vi "DB5000.X写 -AllRest.vi"(0 "引用":refnum<k24>, 5 "semaphore":T1 caption="信号量", 7 "地址名称":string(combo)="字符识别启动信号-读", 11 "error in (no error)":errorcluster caption="错误输入（无错误）") -> (4 "引用输出":refnum<k24>, 15 "error out":errorcluster caption="错误输出")   [LabVIEW 2017]
panel:
  # "字符识别启动信号-读                 DB5000,X00\n电脑1扫码枪触发-读                  DB5000,X100\n电脑1CCD读取字符触发-读         DB5000.101\n电脑1表面检测触发-读               DB5000.102\n电脑1穿管检测触发-读               DB5000.103\n区间位置1-读       DB5000.104\n区间位置2-读       DB5000.105\n区间位置3-读       DB5000.106\n区间位置4-读       DB5000.107\n区间位置5-读       DB5000.108\n区间位置6-读       DB5000.109\n区间位置7-读       DB5000.110\n区间位置8-读       DB5000.111\n区间位置9-读       DB5000.112\n区间位置10-读     DB5000.113\n区间位置11-读      DB5000.114\n区间位置12-读      DB5000.115\n区间位置13-读      DB5000.116\n区间位置14-读      DB5000.117\n区间位置15-读      DB5000.118\n区间位置16-读      DB5000.119\n区间位置17-读      DB5000.120\n区间位置18-读      DB5000.121\n区间位置19-读      DB5000.122\n夹爪1状态-读        DB5000.123\n夹爪2状态-读        DB5000.124\n夹爪3状态-读        DB5000.125\n夹爪4状态-读        DB5000.126\n夹爪5状态-读        DB5000.127\n夹爪6状态-读        DB5000.128\n夹爪7状态-读        DB5000.129\n夹爪8状态-读        DB5000.130\n夹爪9状态-读        DB5000.131\n夹爪10状态-读      DB5000.132\n电脑1产品前后位置切换触发-读       DB5000.133\n电脑1压力获取触发-读                    DB5000.134\nPC1 ready-写                       DB5000.200\n混料-写                               DB5000.201\n字符1检测pass-写                DB5000.202\n字符1检测fail-写                  DB5000.203\n表面检测pass-写                 DB5000.204\n表面检测fail-写                    DB5000.205\n穿管检测pass-写                 DB5000.206\n穿管检测fail-写                    DB5000.207\n扫码枪pass-写                     DB5000.208\n扫码枪fail-写                       DB5000.209\n产品尺寸A-写                      DB5000.210\n产品尺寸B-写                       DB5000.211\n数据传递信号-读                  DB5000.212\n表面检测完成信号-读             DB5000.213\n穿管NG停止信号-写              DB5000.214\n电脑1返工信号-写                 DB5000.215\nPLC初始化信号-读                DB5000.216\n产品尺寸C-写                       DB5000.217\n表面检测错位气缸-读             DB5000.218   \n电脑1衬丝检测触发-读           DB5000.219\n衬丝能检测pass-写               DB5000.220\n衬丝能检测fail-写                  DB5000.221\n长衬丝-写                            DB5000.222\n短衬丝-写                            DB5000.223\n细料-写                              DB5000.225\n粗料-写                              DB5000.226\n一致性检测触发-读               DB5000.227"
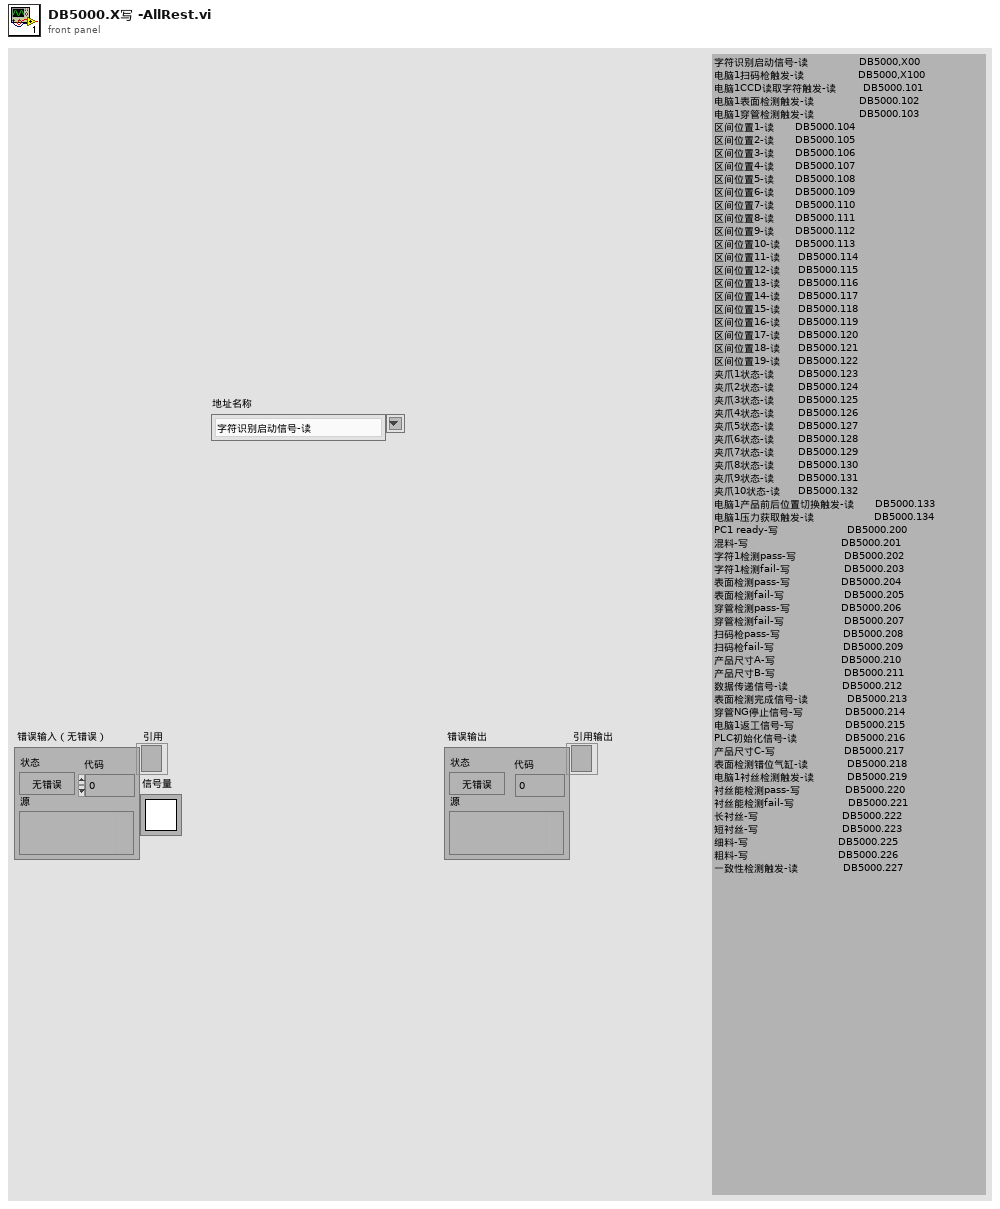
[diagram p1: front panel]
types:
  T1 = typedef "Semaphore RefNum" = refnum<k1>
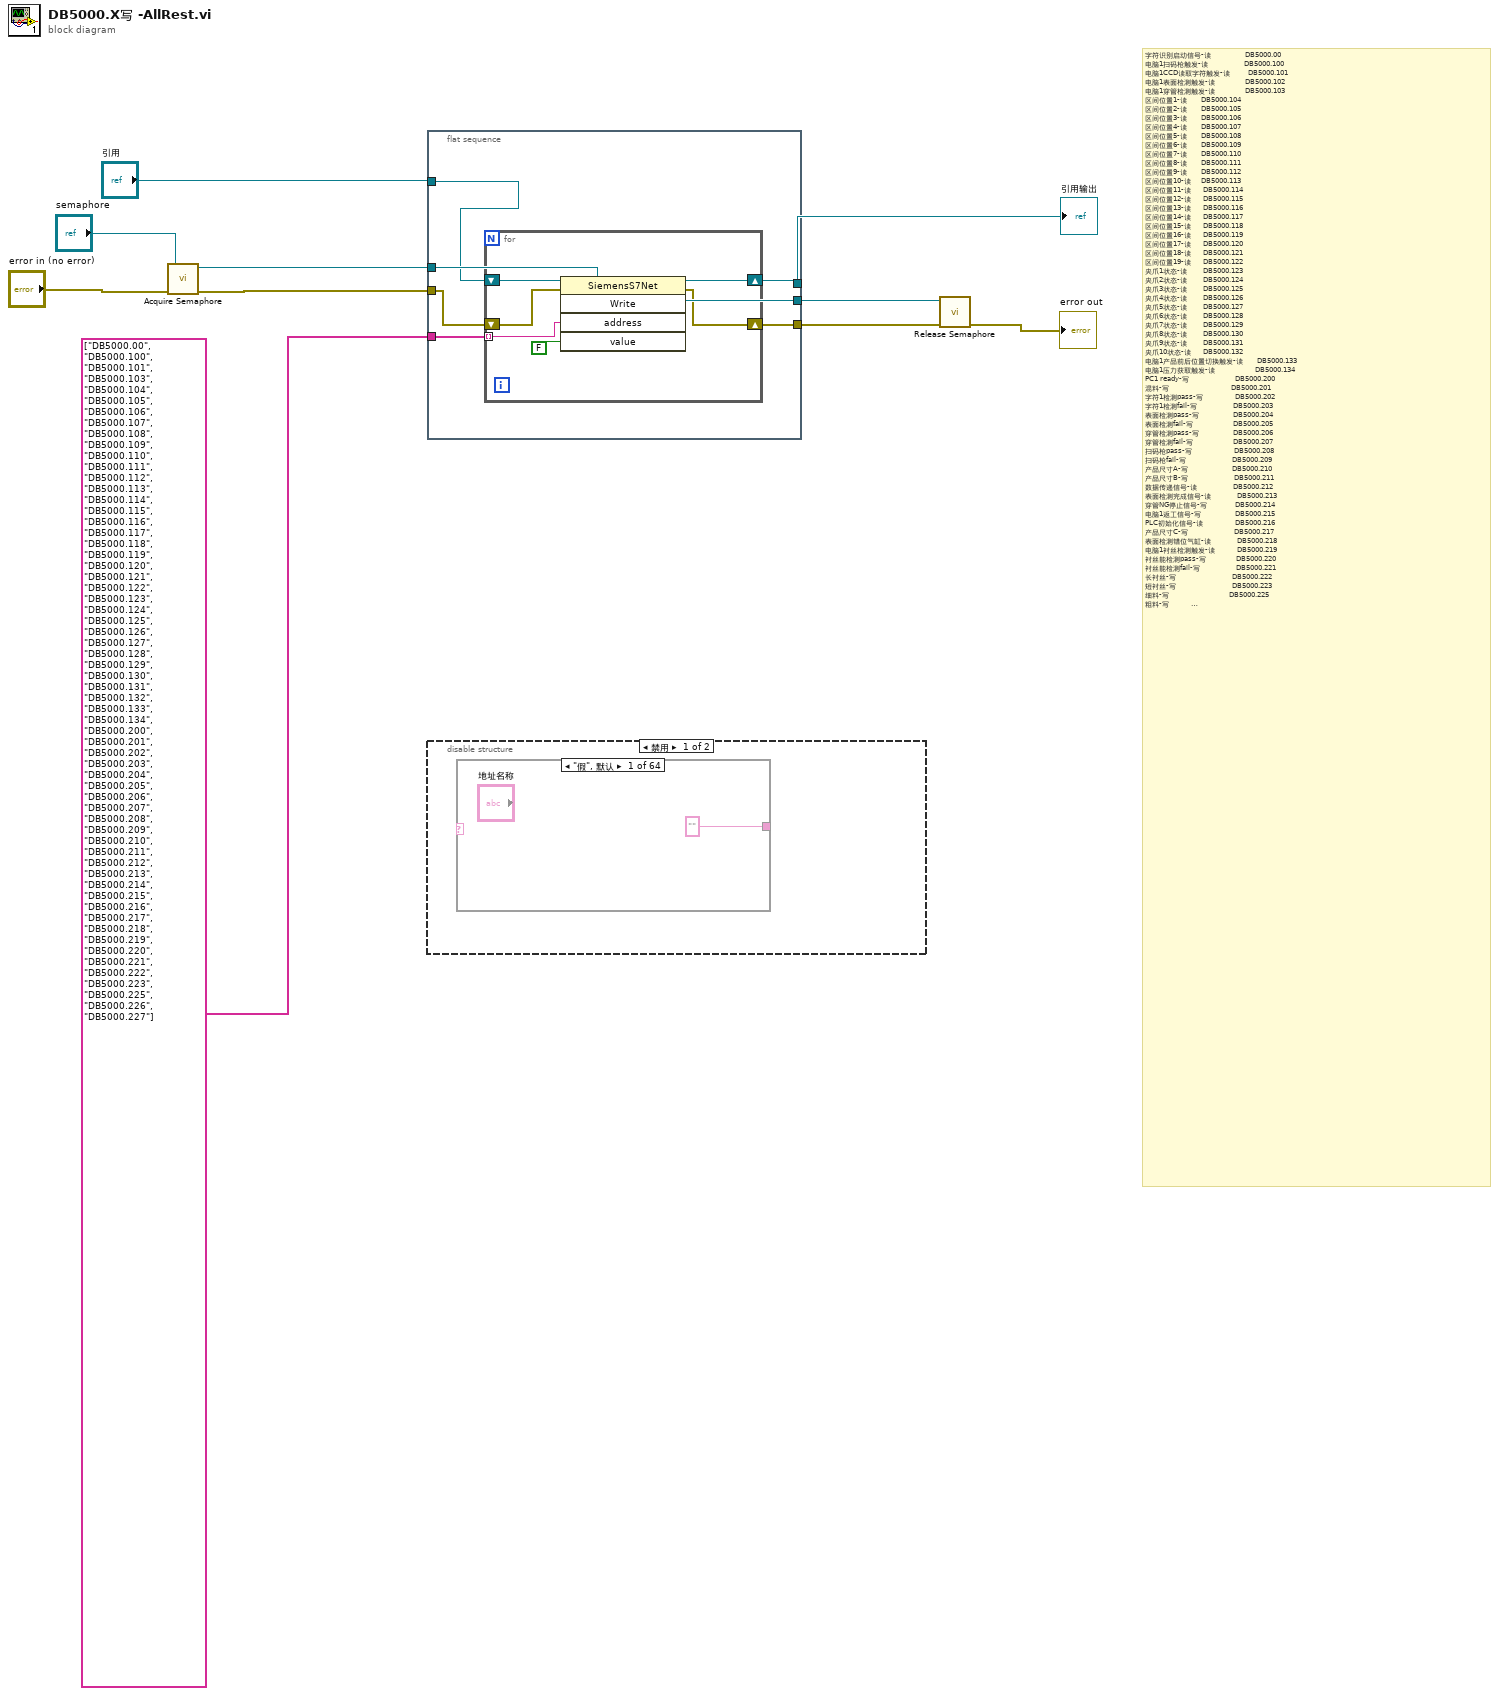
[diagram p0: block diagram]
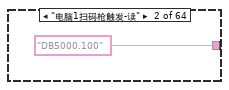
[diagram p2: hidden frame]
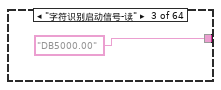
[diagram p3: hidden frame]
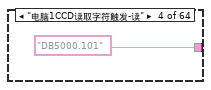
[diagram p4: hidden frame]
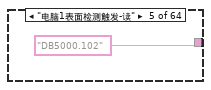
[diagram p5: hidden frame]
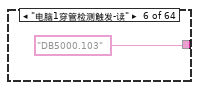
[diagram p6: hidden frame]
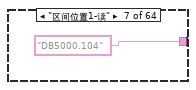
[diagram p7: hidden frame]
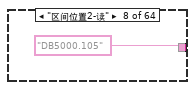
[diagram p8: hidden frame]
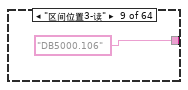
[diagram p9: hidden frame]
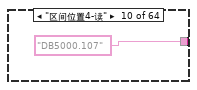
[diagram p10: hidden frame]
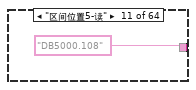
[diagram p11: hidden frame]
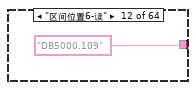
[diagram p12: hidden frame]
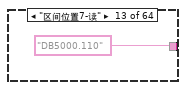
[diagram p13: hidden frame]
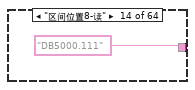
[diagram p14: hidden frame]
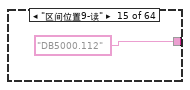
[diagram p15: hidden frame]
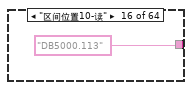
[diagram p16: hidden frame]
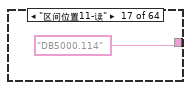
[diagram p17: hidden frame]
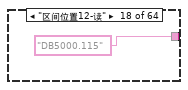
[diagram p18: hidden frame]
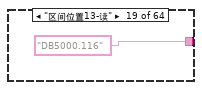
[diagram p19: hidden frame]
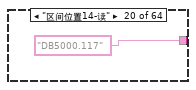
[diagram p20: hidden frame]
diagram:
  # "字符识别启动信号-读                 DB5000.00\n电脑1扫码枪触发-读                  DB5000.100\n电脑1CCD读取字符触发-读         DB5000.101\n电脑1表面检测触发-读               DB5000.102\n电脑1穿管检测触发-读               DB5000.103\n区间位置1-读       DB5000.104\n区间位置2-读       DB5000.105\n区间位置3-读       DB5000.106\n区间位置4-读       DB5000.107\n区间位置5-读       DB5000.108\n区间位置6-读       DB5000.109\n区间位置7-读       DB5000.110\n区间位置8-读       DB5000.111\n区间位置9-读       DB5000.112\n区间位置10-读     DB5000.113\n区间位置11-读      DB5000.114\n区间位置12-读      DB5000.115\n区间位置13-读      DB5000.116\n区间位置14-读      DB5000.117\n区间位置15-读      DB5000.118\n区间位置16-读      DB5000.119\n区间位置17-读      DB5000.120\n区间位置18-读      DB5000.121\n区间位置19-读      DB5000.122\n夹爪1状态-读        DB5000.123\n夹爪2状态-读        DB5000.124\n夹爪3状态-读        DB5000.125\n夹爪4状态-读        DB5000.126\n夹爪5状态-读        DB5000.127\n夹爪6状态-读        DB5000.128\n夹爪7状态-读        DB5000.129\n夹爪8状态-读        DB5000.130\n夹爪9状态-读        DB5000.131\n夹爪10状态-读      DB5000.132\n电脑1产品前后位置切换触发-读       DB5000.133\n电脑1压力获取触发-读                    DB5000.134\nPC1 ready-写                       DB5000.200\n混料-写                               DB5000.201\n字符1检测pass-写                DB5000.202\n字符1检测fail-写                  DB5000.203\n表面检测pass-写                 DB5000.204\n表面检测fail-写                    DB5000.205\n穿管检测pass-写                 DB5000.206\n穿管检测fail-写                    DB5000.207\n扫码枪pass-写                     DB5000.208\n扫码枪fail-写                       DB5000.209\n产品尺寸A-写                      DB5000.210\n产品尺寸B-写                       DB5000.211\n数据传递信号-读                  DB5000.212\n表面检测完成信号-读             DB5000.213\n穿管NG停止信号-写              DB5000.214\n电脑1返工信号-写                 DB5000.215\nPLC初始化信号-读                DB5000.216\n产品尺寸C-写                       DB5000.217\n表面检测错位气缸-读             DB5000.218   \n电脑1衬丝检测触发-读           DB5000.219\n衬丝能检测pass-写               DB5000.220\n衬丝能检测fail-写                  DB5000.221\n长衬丝-写                            DB5000.222\n短衬丝-写                            DB5000.223\n细料-写                              DB5000.225\n粗料-写                              DB5000.226\n一致性检测触发-读               DB5000.227"
  n1 = call <vilib>:"Acquire Semaphore.vi"("error in (no error)"="error in (no error)", "semaphore"="semaphore") -> ("error out"=w9:errorcluster, "semaphore out"=w7:T1)  [unwired: 3 in, 1 out]
  n2 = flat-sequence {
    tunnel: [w16] -> w10
    tunnel: w9 -> [w15]
    tunnel: [w14] -> w8
    tunnel: w7 -> [w14]
    tunnel: "引用" -> [w13]
    tunnel: [w12] -> w2
    tunnel: string[] ["DB5000.00", "DB5000.100", "DB5000.101", "DB5000.103", "DB5000.104", "DB5000.105", "DB5000.106", "DB5000.107", "DB5000.108", "DB5000.109", "DB5000.110", "DB5000.111", "DB5000.112", "DB5000.113", "DB5000.114", "DB5000.115", "DB5000.116", "DB5000.117", "DB5000.118", "DB5000.119", "DB5000.120", "DB5000.121", "DB5000.122", "DB5000.123", "DB5000.124", "DB5000.125", "DB5000.126", "DB5000.127", "DB5000.128", "DB5000.129", "DB5000.130", "DB5000.131", "DB5000.132", "DB5000.133", "DB5000.134", "DB5000.200", "DB5000.201", "DB5000.202", "DB5000.203", "DB5000.204", "DB5000.205", "DB5000.206", "DB5000.207", "DB5000.208", "DB5000.209", "DB5000.210", "DB5000.211", "DB5000.212", "DB5000.213", "DB5000.214", "DB5000.215", "DB5000.216", "DB5000.217", "DB5000.218", "DB5000.219", "DB5000.220", "DB5000.221", "DB5000.222", "DB5000.223", "DB5000.225", "DB5000.226", "DB5000.227"] -> [w11]
    frame #0 {
      n3 = for {
        shift-right: [w22] -> w16
        shift-left: w15 -> [w21]
        shift-right: [w19] -> w12
        shift-left: w13 -> [w20]
        tunnel: w11 -> [w17] mode=indexing
        n4 = invoke class="SiemensS7Net" method="Write"(reference=w20, error in=w21, "address"=w17, "value"=FALSE) -> (reference out=w19:refnum<k24>, error out=w22:errorcluster)  [unwired: 1 in, 3 out]
      }
    }
  }
  n5 = disable-structure shown="禁用" {
    frame Disabled {
      n6 = case shown="\"假\", 默认" {
        selector: _ -> [_ _ _ _ _ _ _ _ _ _ _ _ _ _ _ _ _ _ _ _ _ _ _ _ _ _ _ _ _ _ _ _ _ _ _ _ _ _ _ _ _ _ _ _ _ _ _ _ _ _ _ _ _ _ _ _ _ _ _ _ _ _ _ _]
        tunnel: ["" ("组合框") "DB5000.100" ("组合框") "DB5000.00" ("组合框") "DB5000.101" ("组合框") "DB5000.102" ("组合框") "DB5000.103" ("组合框") "DB5000.104" ("组合框") "DB5000.105" ("组合框") "DB5000.106" ("组合框") "DB5000.107" ("组合框") "DB5000.108" ("组合框") "DB5000.109" ("组合框") "DB5000.110" ("组合框") "DB5000.111" ("组合框") "DB5000.112" ("组合框") "DB5000.113" ("组合框") "DB5000.114" ("组合框") "DB5000.115" ("组合框") "DB5000.116" ("组合框") "DB5000.117" ("组合框") "DB5000.118" ("组合框") "DB5000.119" ("组合框") "DB5000.120" ("组合框") "DB5000.121" ("组合框") "DB5000.122" ("组合框") "DB5000.123" ("组合框") "DB5000.124" ("组合框") "DB5000.125" ("组合框") "DB5000.126" ("组合框") "DB5000.127" ("组合框") "DB5000.128" ("组合框") "DB5000.129" ("组合框") "DB5000.130" ("组合框") "DB5000.131" ("组合框") "DB5000.132" ("组合框") "DB5000.133" ("组合框") "DB5000.134" ("组合框") "DB5000.200" ("组合框") "DB5000.201" ("组合框") "DB5000.202" ("组合框") "DB5000.203" ("组合框") "DB5000.204" ("组合框") "DB5000.205" ("组合框") "DB5000.206" ("组合框") "DB5000.207" ("组合框") "DB5000.208" ("组合框") "DB5000.209" ("组合框") "DB5000.210" ("组合框") "DB5000.211" ("组合框") "DB5000.212" ("组合框") "DB5000.213" ("组合框") "DB5000.214" ("组合框") "DB5000.215" ("组合框") "DB5000.216" ("组合框") "DB5000.217" ("组合框") "DB5000.218" ("组合框") "DB5000.219" ("组合框") "DB5000.220" ("组合框") "DB5000.221" ("组合框") "DB5000.222" ("组合框") "DB5000.223" ("组合框") "DB5000.225" ("组合框") "DB5000.226" ("组合框") "DB5000.227" ("组合框")] -> _
        frame "假", Default {
        }
        frame "电脑1扫码枪触发-读" {
        }
        frame "字符识别启动信号-读" {
        }
        frame "电脑1CCD读取字符触发-读" {
        }
        frame "电脑1表面检测触发-读" {
        }
        frame "电脑1穿管检测触发-读" {
        }
        frame "区间位置1-读" {
        }
        frame "区间位置2-读" {
        }
        frame "区间位置3-读" {
        }
        frame "区间位置4-读" {
        }
        frame "区间位置5-读" {
        }
        frame "区间位置6-读" {
        }
        frame "区间位置7-读" {
        }
        frame "区间位置8-读" {
        }
        frame "区间位置9-读" {
        }
        frame "区间位置10-读" {
        }
        frame "区间位置11-读" {
        }
        frame "区间位置12-读" {
        }
        frame "区间位置13-读" {
        }
        frame "区间位置14-读" {
        }
        frame "区间位置15-读" {
        }
        frame "区间位置16-读" {
        }
        frame "区间位置17-读" {
        }
        frame "区间位置18-读" {
        }
        frame "区间位置19-读" {
        }
        frame "夹爪1状态-读" {
        }
        frame "夹爪2状态-读" {
        }
        frame "夹爪3状态-读" {
        }
        frame "夹爪4状态-读" {
        }
        frame "夹爪5状态-读" {
        }
        frame "夹爪6状态-读" {
        }
        frame "夹爪7状态-读" {
        }
        frame "夹爪8状态-读" {
        }
        frame "夹爪9状态-读" {
        }
        frame "夹爪10状态-读" {
        }
        frame "电脑1产品前后位置切换触发-读" {
        }
        frame "电脑1压力获取触发-读" {
        }
        frame "PC1 ready-写" {
        }
        frame "混料-写" {
        }
        frame "字符1检测pass-写" {
        }
        frame "字符1检测fail-写" {
        }
        frame "表面检测pass-写" {
        }
        frame "表面检测fail-写" {
        }
        frame "穿管检测pass-写" {
        }
        frame "穿管检测fail-写" {
        }
        frame "扫码枪pass-写" {
        }
        frame "扫码枪fail-写" {
        }
        frame "产品尺寸A-写" {
        }
        frame "产品尺寸B-写" {
        }
        frame "数据传递信号-读" {
        }
        frame "表面检测完成信号-读" {
        }
        frame "穿管NG停止信号-写" {
        }
        frame "电脑1返工信号-写" {
        }
        frame "PLC初始化信号-读" {
        }
        frame "产品尺寸C-写" {
        }
        frame "表面检测错位气缸-读" {
        }
        frame "电脑1衬丝检测触发-读" {
        }
        frame "衬丝能检测pass-写" {
        }
        frame "衬丝能检测fail-写" {
        }
        frame "长衬丝-写" {
        }
        frame "短衬丝-写" {
        }
        frame "细料-写" {
        }
        frame "粗料-写" {
        }
        frame "一致性检测触发-读" {
        }
      }
    }
    frame Enabled {
    }
  }
  n7 = call <vilib>:"Release Semaphore.vi"("error in (no error)"=w10, "semaphore"=w8) -> ("error out"=→"error out":errorcluster)  [unwired: 4 in, 1 out]
  "引用输出" <- w2
